vi "inch_to_mm.vi"(1 "inches":sgl format="%#.1f") -> (0 "mm":sgl format="%#.1f")   [LabVIEW 2013]
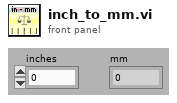
[diagram p1: front panel]
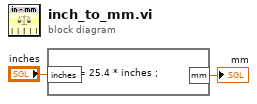
[diagram p0: block diagram]
diagram:
  n1 = formula code="mm = 25.4 * inches ;"("inches"="inches") -> ("mm"=→"mm":dbl)
